vi "Destroy.vi"(7 "Type Specifier":refnum<class>, 8 "error in (no error)":errorcluster, 10 "Force? (f)":bool, 11 "InstrPtr in":refnum<class "InstrPtr.lvclass">) -> (0 "error out":errorcluster, 3 "final Instrument":refnum<class>)   [LabVIEW 2017, in "InstrPtr.lvclass"]
doc: "Finalizes and destroys this Instrument pointer. You can optionally force if some other process still has a handle."
uses:
  InstrPtr.lvclass
  InstrPtr.lvclass/InstrPtr.ctl
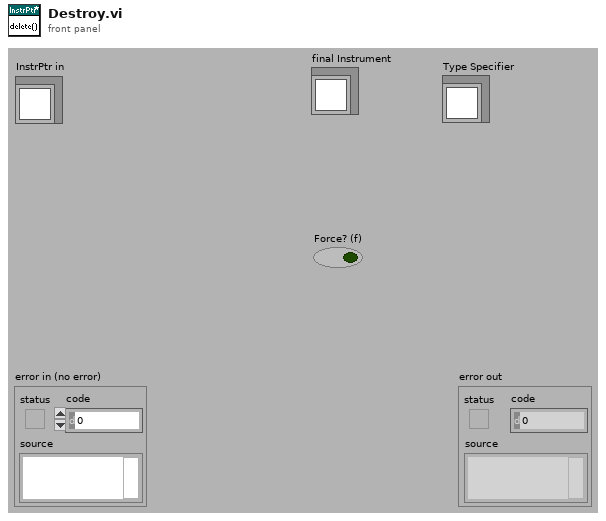
[diagram p1: front panel]
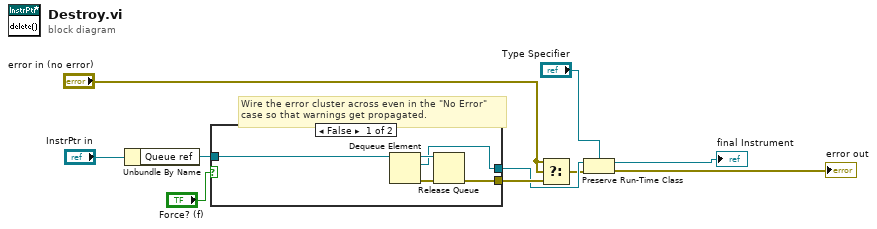
[diagram p0: block diagram]
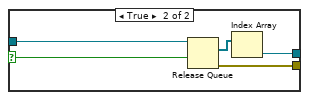
[diagram p2: hidden frame]
diagram:
  # "Wire the error cluster across even in the \"No Error\"\ncase so that warnings get propagated."
  n1 = Unbundle By Name("InstrPtr in") -> ("Queue ref"=w6:refnum<queue>)
  n2 = case shown="False" "Force? (f)" {
    selector: "Force? (f)" -> [_ w16]
    tunnel: w6 -> [w15 w18]
    tunnel: [w12 w20] -> w5
    tunnel: [w11 w17] -> w4
    frame False {
      n3 = Dequeue Element(queue=w15) -> (queue out=w13:refnum<queue>, element=w11:refnum<class>, error out=w14:errorcluster)  [unwired: 1 in, 2 out]
      n4 = Release Queue(queue=w13, error in (no error)=w14) -> (error out=w12:errorcluster)  [unwired: 3 out]
    }
    frame True {
      n5 = Release Queue(queue=w18, force destroy? (F)=w16) -> (remaining elements=w19:refnum<class>[], error out=w20:errorcluster)  [unwired: 1 in, 1 out]
      n6 = Index Array(array=w19) -> (element=w17:refnum<class>)  [unwired: 1 in]
    }
  }
  n7 = Select(t="error in (no error)", s="error in (no error)", f=w5) -> (s? t:f=w1:errorcluster)
  n8 = Preserve Run-Time Class(object in=w4, error in=w1, 2:"Type Specifier") -> (object out=→"final Instrument":refnum<class>, error out=→"error out":errorcluster)
